vi "Better mouse piezo.vi"() -> ()   [LabVIEW 2012]
uses:
  <vilib>/Platform/TimedLoop/XDataNode/timing_clust.ctl
  <vilib>/Platform/TimedLoop/XDataNode/nitl_modes.ctl
  <vilib>/Platform/TimedLoop/XDataNode/wakeup.ctl
  <vilib>/Platform/TimedLoop/XDataNode/XDataNode.xnode
  Program Files/Mad City Labs/NanoDrive/Labview Examples/Madlib.dll
  <vilib>/Platform/TimedLoop/XDataNode/XDNodeRunTimeDep.lvlib
panel:
  in  "stop":bool
  out "Current Z Position (um) 2":dbl format="%.2f"
  out "Current Y Position (um) 2":dbl format="%.2f"
  out "Current X Position (um) 2":dbl format="%.2f"
  in  "Desired Z Position 2":dbl=100.0 min=0.0 max=200.0 step=0.1 format="%.4f"
  in  "Desired Y Position 2":dbl=100.0 min=0.0 max=200.0 step=0.1 format="%.4f"
  in  "Desire X Position 2":dbl=100.0 min=0.0 max=200.0 step=0.1 format="%.4f"
  in  "Handle 2":i32
  # "This example commands the nanopositioner to move to a position,\nwaits a period of time for the nanopositioner to arrive at the position,\nand then reads the position of the  nanopositioner."
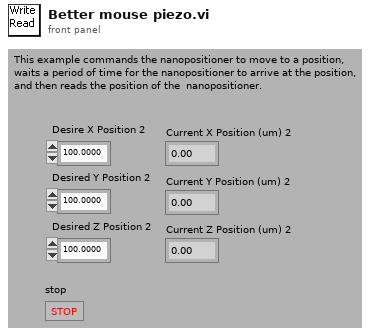
[diagram p1: front panel]
types:
  T1 = typedef "XDNodeRunTimeDep.lvlib/timing_clust.ctl" = cluster{"Expected End [f-1]":u64, "Actual End [f-1]":u64, "Finished Late? [f-1]":bool, "Expected End [i-1]":u64, "Actual End [i-1]":u64, "Finished Late? [i-1]":bool, "Expected Start [i]":u64, "Actual Start [i]":u64, "Expected Start [f]":u64, "Actual Start [f]":u64, "Source Name":string, "Structure Name":string, "Period":i64, "Deadline":i64, "Offset":i64, "Start":i64, "Priority":i32, "Timeout":i32, "Mode":T2, "Wakeup Reason":T3, "Error":errorcluster, "Source Type":string, "Secondary Source Type":string, "Global End Time":u64, "Global Start Time":u64, "Frame Duration":u64, "Iteration Duration":u64, "Assigned CPU":i32, "I/O Scan Engine Mode":u32}
  T2 = typedef "XDNodeRunTimeDep.lvlib/nitl_modes.ctl" = enum32{"No Change", "Process missed periods, maintain original phase", "Discard missed periods, maintain original phase", "Process missed periods, ignore original phase", "Discard missed periods, ignore original phase"}
  T3 = typedef "XDNodeRunTimeDep.lvlib/wakeup.ctl" = enum32{"Normal", "Aborted", "Asynchronous wakeup", "Timing source error", "Timed loop error", "Timeout"}
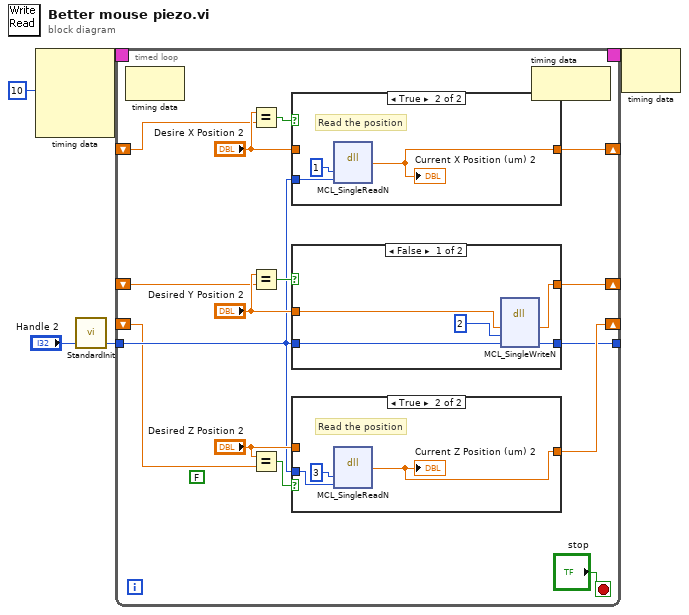
[diagram p0: block diagram]
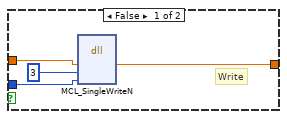
[diagram p2: hidden frame]
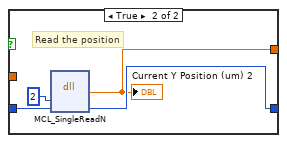
[diagram p3: hidden frame]
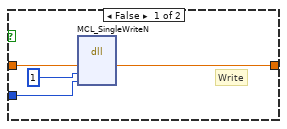
[diagram p4: hidden frame]
diagram:
  n1 = node-c288(10 ("Period")) -> (w5:T1)  [unwired: 3 out]
  n2 = call "StandardInit.vi"("Incoming Handle"="Handle 2") -> ("Outgoing Handle"=w1:i32)
  n3 = timed-loop {
    tunnel: w1 -> [w14]
    tunnel: [w10] -> _
    shift-right: [w13] -> _
    shift-left: _ -> [w7]
    shift-right: [w12] -> _
    shift-left: _ -> [w8]
    shift-right: [w11] -> _
    shift-left: _ -> [w9]
    timing: w5 -> [_]
    timing-out: [_] -> w4
    stop <- "stop" stop-if-true
    (unwired) FALSE
    n4 = node-c288() -> ()  [unwired: 2 out]
    n5 = Equal?(x="Desire X Position 2", y=w7) -> (x = y?=w19:bool)
    n6 = Equal?(x="Desired Y Position 2", y=w8) -> (x = y?=w17:bool)
    n7 = Equal?(x="Desired Z Position 2", y=w9) -> (x = y?=w15:bool)
    n8 = case shown="True" w19 {
      tunnel: w14 -> [w40 w45]
      tunnel: [w39 w44] -> w13
      tunnel: "Desire X Position 2" -> [w41 _]
      frame False {
        # "Write"
        n9 = dll-call lib="C:/Program Files/Mad City Labs/NanoDrive/Labview Examples/Madlib.dll" fn="MCL_SingleWriteN"("position"=w41, "axis"=u32 1, "handle"=w40) -> ("position"=w39:dbl)  [unwired: 5 in, 3 out]
      }
      frame True {
        # "Read the position"
        n10 = dll-call lib="C:/Program Files/Mad City Labs/NanoDrive/Labview Examples/Madlib.dll" fn="MCL_SingleReadN"("axis"=u32 1, "handle"=w45) -> (w44:dbl)  [unwired: 5 in, 2 out]
        "Current X Position (um) 2" <- w44
      }
    }
    n11 = case shown="False" w17 {
      tunnel: [w30 w38] -> w10
      tunnel: w14 -> [w32 w37]
      tunnel: [w31 w36] -> w12
      tunnel: "Desired Y Position 2" -> [w33 _]
      frame False {
        n12 = dll-call lib="C:/Program Files/Mad City Labs/NanoDrive/Labview Examples/Madlib.dll" fn="MCL_SingleWriteN"("position"=w33, "axis"=u32 2, "handle"=w32) -> ("position"=w31:dbl, "handle"=w30:i32)  [unwired: 4 in, 3 out]
      }
      frame True {
        # "Read the position"
        n13 = dll-call lib="C:/Program Files/Mad City Labs/NanoDrive/Labview Examples/Madlib.dll" fn="MCL_SingleReadN"("axis"=u32 2, "handle"=w37) -> (w36:dbl, "handle"=w38:i32)  [unwired: 4 in, 2 out]
        "Current Y Position (um) 2" <- w36
      }
    }
    n14 = case shown="True" w15 {
      tunnel: w14 -> [w23 w29]
      tunnel: [w24 w28] -> w11
      tunnel: "Desired Z Position 2" -> [w25 _]
      frame False {
        # "Write"
        n15 = dll-call lib="C:/Program Files/Mad City Labs/NanoDrive/Labview Examples/Madlib.dll" fn="MCL_SingleWriteN"("position"=w25, "axis"=u32 3, "handle"=w23) -> ("position"=w24:dbl)  [unwired: 5 in, 3 out]
      }
      frame True {
        # "Read the position"
        n16 = dll-call lib="C:/Program Files/Mad City Labs/NanoDrive/Labview Examples/Madlib.dll" fn="MCL_SingleReadN"("axis"=u32 3, "handle"=w29) -> ("return type"=w28:dbl)  [unwired: 5 in, 2 out]
        "Current Z Position (um) 2" <- w28
      }
    }
    n17 = node-c288() -> ()  [unwired: 2 out]
  }
  n18 = node-c288(w4) -> ()  [unwired: 1 out]
